vi "Read OfficeTron3000.vi"(11 "OT3IPrinter In":refnum<class "OT3IPrinter.lvclass">) -> (2 "OfficeTron3000":refnum<class "OfficeTron3000.lvclass">, 3 "OT3IPrinter Out":refnum<class "OT3IPrinter.lvclass">)   [LabVIEW 2018, in "OfficeTron3000.lvlib" / "OT3IPrinter.lvclass"]
uses:
  OT3IPrinter.lvclass
  OfficeTron3000/OfficeTron3000.lvclass
  OT3IPrinter.lvclass/OT3IPrinter.ctl
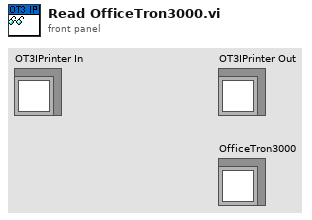
[diagram p1: front panel]
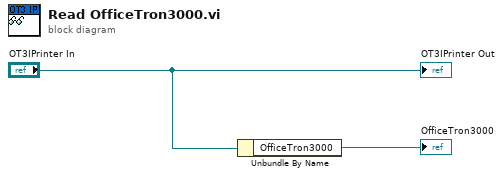
[diagram p0: block diagram]
diagram:
  n1 = Unbundle By Name("OT3IPrinter In") -> ("OfficeTron3000"=→"OfficeTron3000":refnum<class "OfficeTron3000.lvclass">)
  "OT3IPrinter Out" <- "OT3IPrinter In"
